vi "RootExists.vi"(11 "path":path) -> (2 "file or folder exists?":bool)   [LabVIEW 2018]
doc: "Checks if root directory (e.g. C:/) exists. Returns boolean true if yes."
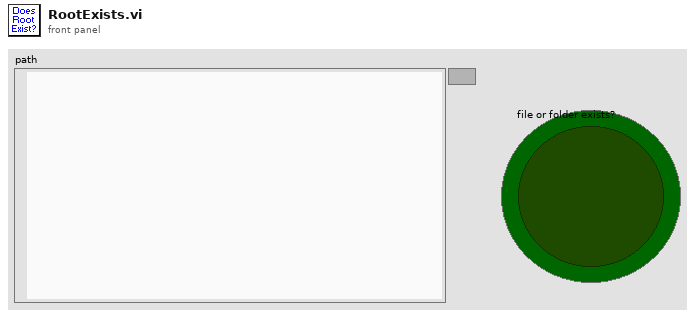
[diagram p1: front panel]
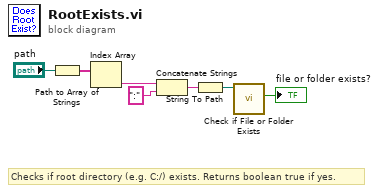
[diagram p0: block diagram]
diagram:
  # "Checks if root directory (e.g. C:/) exists. Returns boolean true if yes."
  n1 = Path to Array of Strings(0:"path") -> (2:w7:string[])  [unwired: 1 out]
  n2 = Index Array(array=w7) -> (element=w2:string)  [unwired: 1 in]
  n3 = Concatenate Strings(w2, ":" ("string")) -> (w1:string)
  n4 = String To Path(string=w1) -> (path=w6:path)
  n5 = call <vilib>:"Check if File or Folder Exists.vi"("path"=w6) -> ("file or folder exists?"=→"file or folder exists?":bool)  [unwired: 8 in, 2 out]
